vi "180 Degree Spin.vi"(4 "Z Axis Input":dbl) -> (1 "Z Axis Output":dbl)   [LabVIEW 2014]
uses:
  180 Degree Spin.ctl
  <vilib>/Rock Robotics/WPI/Joystick/WPI_JoystickGetSetRefNum.vi
  Gyro/Gyro Angle.vi
  <vilib>/addons/control/pid/pid.llb/PID (DBL).vi
  <vilib>/addons/control/pid/NI_PID_pid.lvlib
panel:
  in  "180 Spin Gains":T1={"proportional gain (Kc)"=1.0, "integral time (Ti, min)"=0.01, "derivative time (Td, min)"=0.0} {"derivative time (Td, min)" format="%.3f"; "integral time (Ti, min)" format="%.3f"; "proportional gain (Kc)" format="%.3f"}
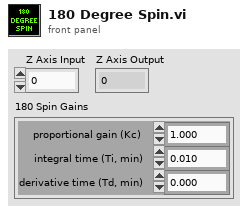
[diagram p1: front panel]
types:
  T1 = cluster{"proportional gain (Kc)":dbl, "integral time (Ti, min)":dbl, "derivative time (Td, min)":dbl}
  T2 = typedef "180 Degree Spin.ctl" = enum16{"WaitingForInput", "GetGyroPosition", "SetPidOnZAxis"}
  T3 = typedef "WPI_I2CDevRef.ctl" = cluster{"DevStatus":errorcluster, "Controller":T4, "Device Address":u8, "Handle":i32, "I2C Bus":T5}
  T4 = typedef "FPGA_TypedefDigitalModule.ctl" = enum16{"Controller 1"}
  T5 = typedef "i2c_bus.ctl" = enum16{"I2C On-Board", "I2C MXP", "Invalid"}
  T6 = typedef "WPI_JoystickDevRef.ctl" = cluster{"Device":T7}
  T7 = typedef "WPI_JoystickDeviceEnum.ctl" = enum16{"USB 0", "USB 1", "USB 2", "USB 3", "USB 4", "USB 5"}
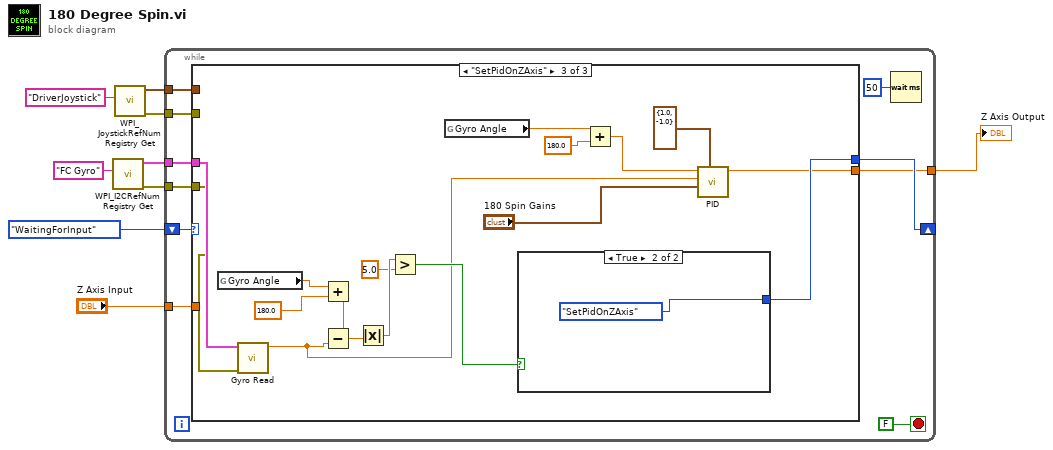
[diagram p0: block diagram]
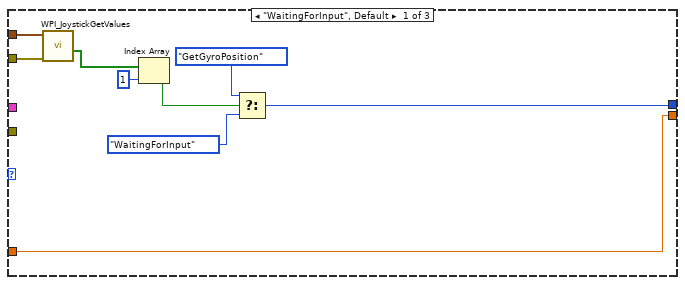
[diagram p2: hidden frame]
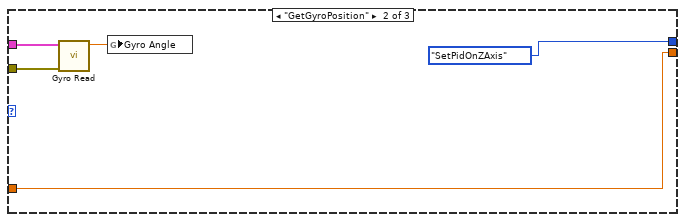
[diagram p3: hidden frame]
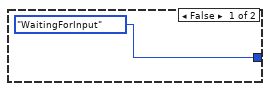
[diagram p4: hidden frame]
diagram:
  n1 = call <vilib>:"WPI_I2CRefNum Registry Get.vi"("refnum name"="FC Gyro") -> ("error out"=w3:errorcluster, "I2CDevRef"=w4:T3)  [unwired: 9 in]
  n2 = call <vilib>:"WPI_JoystickRefNum Registry Get.vi"("refnum name"="DriverJoystick") -> ("error out"=w6:errorcluster, "JoystickDevRef"=w7:T6)  [unwired: 9 in]
  n3 = while {
    tunnel: w7 -> [w16]
    tunnel: w6 -> [w15]
    tunnel: w4 -> [w14]
    tunnel: w3 -> [w13]
    shift-right: [w12] -> _
    shift-left: 180_Degree_Spin."WaitingForInput" ("180 Spin") -> [w17]
    tunnel: [w11] -> w2
    tunnel: "Z Axis Input" -> [w10]
    stop <- FALSE stop-if-true
    n4 = case shown="\"SetPidOnZAxis\"" w17 {
      tunnel: w16 -> [w28 _ _]
      tunnel: w15 -> [w27 _ _]
      tunnel: w14 -> [_ w31 w37]
      tunnel: w13 -> [_ w30 w36]
      tunnel: [w21 180_Degree_Spin."SetPidOnZAxis" ("180 Spin") w43] -> w12
      tunnel: [w20 w29 w34] -> w11
      tunnel: w10 -> [w20 w29 _]
      frame "WaitingForInput", Default {
        n5 = call <vilib>:"WPI_JoystickGetValues.vi"("error in (no error)"=w27, "JoystickDevRef"=w28) -> ("Buttons"=w26:bool[])  [unwired: 5 in, 4 out]
        n6 = Index Array(array=w26, index=1) -> (element=w24:bool)
        n7 = Select(t=180_Degree_Spin."GetGyroPosition" ("180 Spin"), s=w24, f=180_Degree_Spin."WaitingForInput" ("180 Spin")) -> (s? t:f=w21:T2)
      }
      frame "GetGyroPosition" {
        n8 = call "Gyro Read.vi"("error in (no error)"=w30, "I2CDevRef In"=w31) -> ("Angle"=w32:dbl)  [unwired: 7 in, 2 out]
        n9 = global write "Gyro Angle.vi" "Gyro Angle"(w32) -> ()
      }
      frame "SetPidOnZAxis" {
        n10 = global read "Gyro Angle.vi" "Gyro Angle"() -> (w50:dbl)
        n11 = call "Gyro Read.vi"("error in (no error)"=w36, "I2CDevRef In"=w37) -> ("Angle"=w35:dbl)  [unwired: 7 in, 2 out]
        n12 = Add(x=w50, y=180.0) -> (x+y=w48:dbl)
        n13 = Subtract(x=w48, y=w35) -> (x-y=w47:dbl)
        n14 = Absolute Value(x=w47) -> (abs(x)=w46:dbl)
        n15 = Greater?(x=w46, y=5.0) -> (0:w44:bool)
        n16 = global read "Gyro Angle.vi" "Gyro Angle"() -> (w38:dbl)
        n17 = case shown="True" w44 {
          tunnel: [180_Degree_Spin."WaitingForInput" ("180 Spin") 180_Degree_Spin."SetPidOnZAxis" ("180 Spin")] -> w43
          frame False {
          }
          frame True {
          }
        }
        n18 = Add(x=w38, y=180.0) -> (x+y=w40:dbl)
        n19 = call-poly <vilib>:"PID.vi"("output range"=cluster{"output high":dbl, "output low":dbl} {"output high"=1.0, "output low"=-1.0}, "PID gains"="180 Spin Gains", "process variable"=w35, "setpoint"=w40) -> ("output"=w34:dbl)  [unwired: 6 in, 1 out]
      }
    }
    n20 = Wait (ms)(milliseconds to wait=u32 50) -> ()  [unwired: 1 out]
  }
  "Z Axis Output" <- w2
